vi "Check for Coil Mapping Conflicts.vi"(8 "error in (no error)":errorcluster, 11 "Coiil Group Ref in":T1 format="%.0x") -> (0 "error out":errorcluster, 1 "Conflicts?":bool, 2 "Conflicts":T2(array[cluster]), 3 "Coil Group Ref out":T1 format="%.0x")   [LabVIEW 2015, in "Modbus Master System Explorer.lvlib"]
uses:
  Modbus Master System Explorer.lvlib
  <vilib>/NI Veristand/Custom Device API/Custom Device Item Ref.ctl
  Modbus Type.ctl
  <vilib>/NI VeriStand/Custom Device API/Custom Device API.lvlib
  Shared/Modbus Master Shared.lvlib
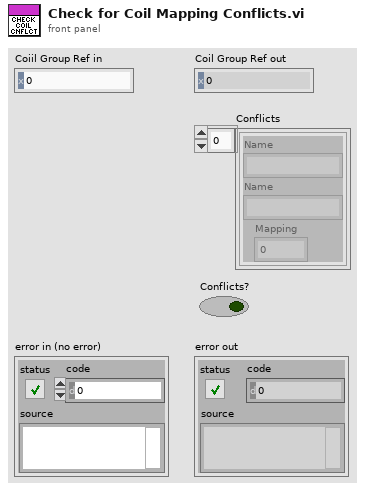
[diagram p1: front panel]
types:
  T1 = typedef "Custom Device API.lvlib/Custom Device Item Ref.ctl" = u64
  T2 = cluster{"Name":string, "Name":string, "Mapping":u16}[]
  T3 = typedef "Modbus Master Shared.lvlib/Modbus Type.ctl" = enum16{"Coil", "Discrete Input", "Holding Register", "Input Register"}
  T4 = typedef "Custom Device API.lvlib/Custom Device Item Info.ctl" = cluster{"Name":string, "Is Channel":bool, "GUID":string, "Is Waveform":bool}
  T5 = cluster{"Name":string, "Name":string, "Mapping":u16}
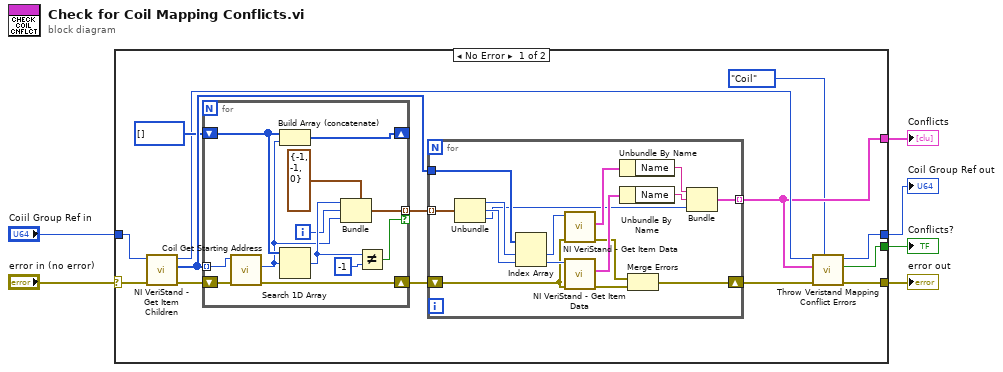
[diagram p0: block diagram]
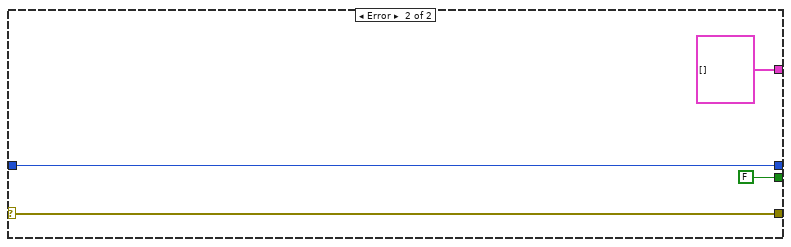
[diagram p2: hidden frame]
diagram:
  n1 = case shown="No Error" "error in (no error)" {
    selector: "error in (no error)" -> [w16 w51]
    tunnel: "Coiil Group Ref in" -> [w17 w52]
    tunnel: [w13 w52] -> w4
    tunnel: [w11 T2 []] -> w3
    tunnel: [w9 w51] -> w2
    tunnel: [w8 FALSE ("Conflicts?")] -> w1
    frame No Error {
      n2 = call <vilib>:"NI VeriStand - Get Item Children.vi"("error in (no error)"=w16, "Item Ref in"=w17) -> ("error out"=w15:errorcluster, "Child Refs"=w20:T1[], "Item Ref out"=w12:T1)  [unwired: 6 in, 1 out]
      n3 = for {
        tunnel: w20 -> [w48] mode=indexing
        shift-right: [w47] -> _
        shift-left: u16[] [] ("Starting Address") -> [w46]
        tunnel: [w43] -> w19 mode=indexing if=w42
        shift-right: [w37] -> w14
        shift-left: w15 -> [w38]
        i -> [w40]
        n4 = call "Coil Get Starting Address.vi"("error in (no error)"=w38, "Item Ref in"=w48) -> ("error out"=w37:errorcluster, "Starting Address"=w39:u16)  [unwired: 7 in, 1 out]
        n5 = Build Array (concatenate)(w46, w39) -> (w47:u16[])
        n6 = Search 1D Array(1D array=w46, element=w39) -> (index of element=w41:i32)  [unwired: 1 in]
        n7 = Bundle(cluster=cluster{"y":i32, "y 2":i32, "Mapping":u16} {"y"=-1, "y 2"=-1, "Mapping"=0} ("Conflicting Indices"), "y"=w41, "y 2"=w40, "Mapping"=w39) -> (w43:cluster{"y":i32, "y 2":i32, "Mapping":u16})
        n8 = Not Equal?(x=w41, y=-1) -> (x != y?=w42:bool)
      }
      n9 = for {
        tunnel: w19 -> [w36] mode=indexing
        tunnel: w20 -> [w35]
        tunnel: [w26] -> w11 mode=indexing
        shift-right: [w21] -> w10
        shift-left: w14 -> [w24]
        n10 = Unbundle(w36) -> ("y"=w34:i32, "y 2"=w33:i32, "Mapping"=w25:u16)
        n11 = Index Array(array=w35, index #1=w34, index #2=w33) -> (element #1=w32:T1, element #2=w31:T1)
        n12 = call <vilib>:"NI VeriStand - Get Item Data.vi"("error in (no error)"=w24, "Item Ref in"=w32) -> ("error out"=w23:errorcluster, "Item Info"=w30:T4)  [unwired: 8 out]
        n13 = call <vilib>:"NI VeriStand - Get Item Data.vi"("error in (no error)"=w24, "Item Ref in"=w31) -> ("error out"=w22:errorcluster, "Item Info"=w29:T4)  [unwired: 8 out]
        n14 = Unbundle By Name(w30) -> ("Name"=w28:string)
        n15 = Unbundle By Name(w29) -> ("Name"=w27:string)
        n16 = Merge Errors(w23, w22) -> (w21:errorcluster)
        n17 = Bundle("Name"=w28, "Name"=w27, "Mapping"=w25) -> (w26:T5)  [unwired: 1 in]
      }
      n18 = call "Throw Veristand Mapping Conflict Errors.vi"("Type"=Modbus_Type."Coil", "error in (no error)"=w10, "Conflicts In"=w11, "Item Ref in"=w12) -> ("error out"=w9:errorcluster, "Conflicts?"=w8:bool, "Node Ref out"=w13:T1)  [unwired: 5 in]
    }
    frame Error {
    }
  }
  "Conflicts?" <- w1
  "Conflicts" <- w3
  "Coil Group Ref out" <- w4
  "error out" <- w2
